vi "GenerateOverriddenSystemDefinition.vi"(8 "error in (no error)":errorcluster, 10 "absolute override file":path[](array[path]), 11 "absolute system definition file":path) -> (0 "error out":errorcluster, 3 "absolute overridden system definition file":path)   [LabVIEW 2015, in "VeriStandTestCase.lvclass"]
uses:
  VeriStandTestCase.lvclass
  <vilib>/xml/Load XML File.vi
  <vilib>/xml/Close Reference(Node).vi
  <vilib>/xml/NI_XML.lvlib
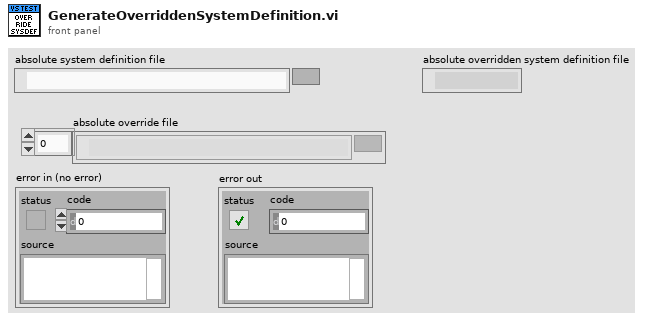
[diagram p1: front panel]
types:
  T1 = cluster{"path":string, "value":string, "encoding":string}[]
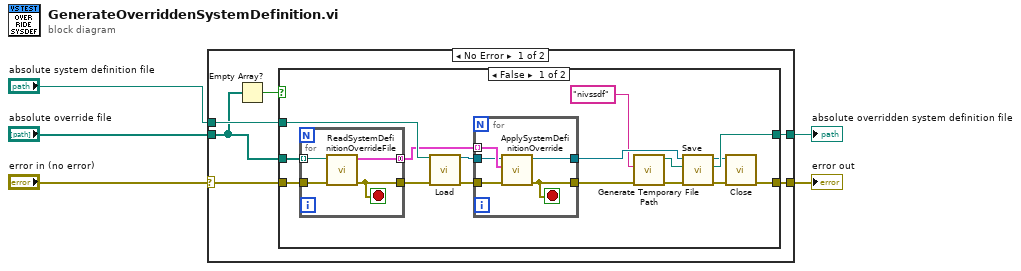
[diagram p0: block diagram]
diagram:
  n1 = case shown="No Error" "error in (no error)" {
    selector: "error in (no error)" -> [w11 w40]
    tunnel: "absolute override file" -> [w7 _]
    tunnel: "absolute system definition file" -> [w10 w39]
    tunnel: [w9 w40] -> w2
    tunnel: [w8 w39] -> w1
    frame No Error {
      n2 = Empty Array?(array=w7) -> (empty?=w6:bool)
      n3 = case shown="False" w6 {
        tunnel: w11 -> [w27 w37]
        tunnel: w10 -> [w26 w38]
        tunnel: [w25 w37] -> w9
        tunnel: [w24 w38] -> w8
        tunnel: w7 -> [w12 _]
        frame False {
          n4 = for {
            tunnel: [w36] -> w23 mode=concatenating
            tunnel: w12 -> [w35] mode=indexing
            tunnel: [w34] -> w21
            tunnel: w27 -> [w33]
            stop <- w34 stop-if-true
            n5 = call "ReadSystemDefinitionOverrideFile.vi"("error in (no error)"=w33, "configuration file path"=w35) -> ("error out"=w34:errorcluster, "override items"=w36:T1)  [unwired: 8 in]
          }
          n6 = call-poly <vilib>:"Load.vi"("path to XML document"=w26, "error in (no error)"=w21) -> ("DOM document out"=w22:refnum<k20>, "error out"=w20:errorcluster)  [unwired: 11 in, 1 out]
          n7 = for {
            tunnel: w23 -> [w32] mode=indexing
            tunnel: w20 -> [w31]
            tunnel: [w30] -> w14
            tunnel: w22 -> [w29]
            tunnel: [w28] -> w17
            stop <- w30 stop-if-true
            n8 = call "ApplySystemDefinitionOverride.vi"("error in (no error)"=w31, "override item"=w32, "node in"=w29) -> ("error out"=w30:errorcluster, "node out"=w28:refnum<k20>)  [unwired: 7 in]
          }
          n9 = call <vilib>:"Generate Temporary File Path.vi"("error in (no error)"=w14, "Temporary File Extension (tmp)"="nivssdf") -> ("error out"=w13:errorcluster, "Unique Temporary File Path"=w15:path)  [unwired: 8 in]
          n10 = call <vilib>:"Save.vi"("error in (no error)"=w13, "XML file path"=w15, "DOM document in"=w17) -> ("error out"=w19:errorcluster, "XML file path out"=w24:path, "DOM document out"=w18:refnum<k20>)  [unwired: 6 in]
          n11 = call-poly <vilib>:"Close.vi"("error in (no error)"=w19, "node"=w18) -> ("error out"=w25:errorcluster)  [unwired: 7 in]
        }
        frame True {
        }
      }
    }
    frame Error {
    }
  }
  "error out" <- w2
  "absolute overridden system definition file" <- w1
